vi "VNA_QueryGP.vi"(5 "Simulation":bool, 7 "HAPS_Equipment":enum16{"Keysight", "R&S"}(ring), 8 "error in":errorcluster) -> (0 "error out":errorcluster, 3 "queryMarker":cluster{"gain":dbl, "phase":dbl} {"phase" format="%#.3f"; "gain" format="%#.3f"})   [LabVIEW 2023, in "HAPS.lvlib"]
uses:
  HAPS.lvlib
  CTL/RS_ZNA.ctl
  CTL/Keysight_VNA.ctl
  Keysight/Keysight.lvlib
  R_S/R_S.lvlib
panel:
  in  "VISA IN":refnum<visa-resource-name>="TCPIP0::192.168.119.45::inst0::INSTR"
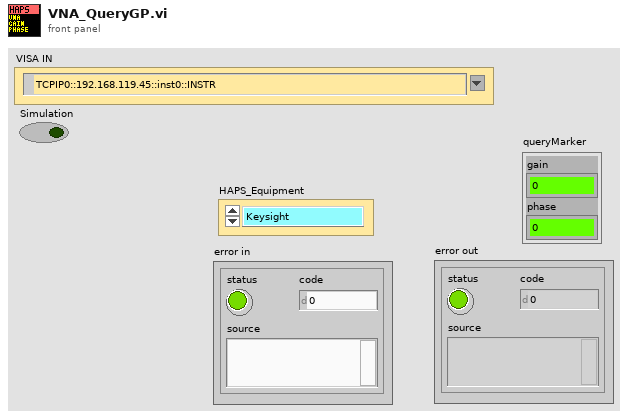
[diagram p1: front panel]
types:
  T1 = typedef "RS_ZNA.ctl" = enum16{"Init", "Close", "set_SweepPoint", "set_MeasFormat", "set_FreqStartStop", "set_MeasPAR_S", "set_MarkerON", "set_MarkerOFF", "set_MarkerFreq", "set_MarkerFormat", "set_TriggerSingle", "query_GainPhase"}
  T2 = typedef "Keysight_VNA.ctl" = enum16{"Init", "queryMarker", "setSweepPoint", "setMarkerFreq", "setMeasureFormat", "setFreqStartStop", "setMarkerOnOFF", "setMarkerFormat_LOGP", "setMeasPAR_S", "setTriggerSingle", "Trigger_Save_SnP", "Trigger_Single", "Close"}
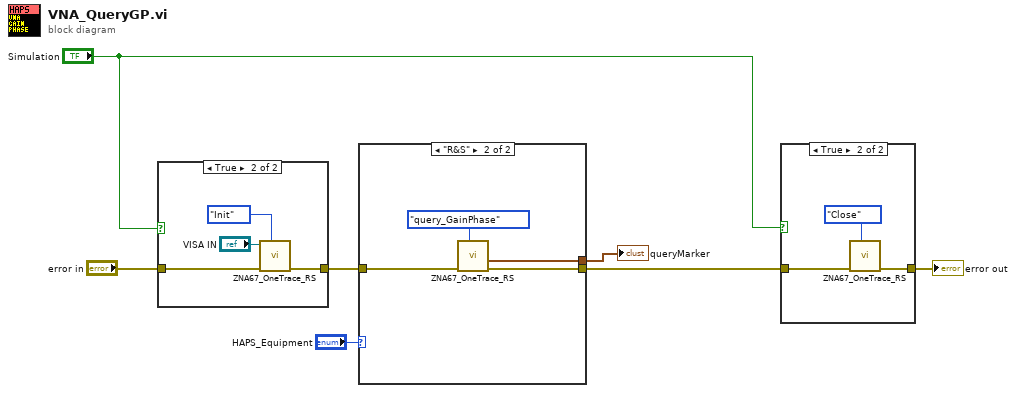
[diagram p0: block diagram]
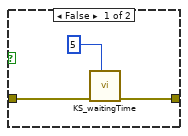
[diagram p3: hidden frame]
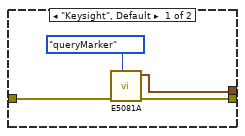
[diagram p4: hidden frame]
diagram:
  n1 = case shown="True" "Simulation" {
    tunnel: "error in" -> [w9 w14]
    tunnel: [w10 w13] -> w4
    frame False {
      n2 = call "KS_waitingTime.vi"("Waiting Time(ms)"=u32 5, "error in"=w9) -> ("error out"=w10:errorcluster)  [unwired: 9 in]
    }
    frame True {
      n3 = call "ZNA67_OneTrace_RS.vi"("ZNA_Func."=RS_ZNA."Init", "error in"=w14, "VISA IN"="VISA IN") -> ("error out"=w13:errorcluster)  [unwired: 5 in, 3 out]
    }
  }
  n4 = case shown="\"R&S\"" "HAPS_Equipment" {
    tunnel: w4 -> [w18 w21]
    tunnel: [w17 w22] -> w3
    tunnel: [w15 w19] -> w6
    frame "Keysight", Default {
      n5 = call "E5081A.vi"("Function_VNA"=Keysight_VNA."queryMarker", "error in"=w18) -> ("error out"=w17:errorcluster, "queryMarker"=w15:cluster{"gain":dbl, "phase":dbl})  [unwired: 8 in]
    }
    frame "R&S" {
      n6 = call "ZNA67_OneTrace_RS.vi"("ZNA_Func."=RS_ZNA."query_GainPhase", "error in"=w21) -> ("error out"=w22:errorcluster, "queryMarker"=w19:cluster{"gain":dbl, "phase":dbl})  [unwired: 6 in, 2 out]
    }
  }
  "queryMarker" <- w6
  n7 = case shown="True" "Simulation" {
    tunnel: w3 -> [w23 w26]
    tunnel: [w23 w25] -> w2
    frame False {
    }
    frame True {
      n8 = call "ZNA67_OneTrace_RS.vi"("ZNA_Func."=RS_ZNA."Close", "error in"=w26) -> ("error out"=w25:errorcluster)  [unwired: 6 in, 3 out]
    }
  }
  "error out" <- w2
